vi "Fuzzy_PID.vi"(1 "下限":dbl=330.0 max=349.0 format="%#_13g", 2 "上限":dbl=346.0 min=321.0, 3 "起始值":dbl) -> (0 "调整值":dbl format="%_6g")   [LabVIEW 2016]
uses:
  <vilib>/addons/control/pid/pid.llb/PID (DBL).vi
  <vilib>/addons/Fuzzy Logic/FL Fuzzy Controller (MIMO).vi
  <vilib>/addons/control/pid/NI_PID_pid.lvlib
  <vilib>/addons/Fuzzy Logic/NI_Fuzzy_Logic_API.lvlib
panel:
  out "波形图表":cluster{dbl, "期望值":dbl}(graph)
  out "输入值":dbl
  out "误差变化率":dbl
  out "误差":dbl
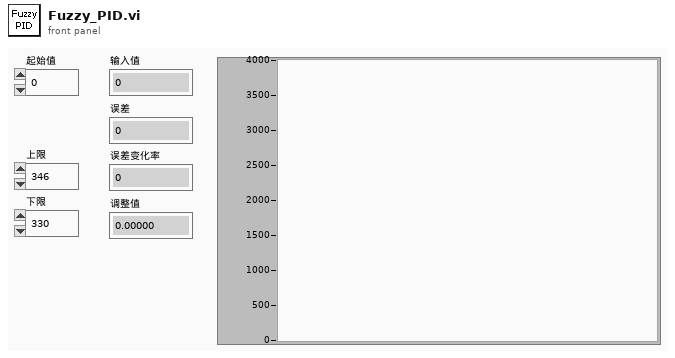
[diagram p1: front panel]
types:
  T1 = typedef "NI_Fuzzy_Logic_API.lvlib/FL System.ctl" = cluster{"input variables":T2[], "output variables":T2[], "rules":T5[], "defuzzification method":T11, "description":string, "user MF interpolating polynomials":T12[]}
  T2 = typedef "NI_Fuzzy_Logic_API.lvlib/FL Variable.ctl" = cluster{"name":string, "range":dbl[], "MFs":T3[]}
  T3 = typedef "NI_Fuzzy_Logic_API.lvlib/FL Membership Function.ctl" = cluster{"name":string, "shape":T4, "points":dbl[], "color":u32, "user-defined shape index":i32}
  T4 = typedef "NI_Fuzzy_Logic_API.lvlib/FL Membership Function Shape.ctl" = u16
  T5 = typedef "NI_Fuzzy_Logic_API.lvlib/FL Rule.ctl" = cluster{"antecedents":T6[], "antecedent connective":T8, "consequents":T9[], "consequent implication":T10, "degree of support":dbl}
  T6 = typedef "NI_Fuzzy_Logic_API.lvlib/FL Antecedent.ctl" = cluster{"Var Index":i32, "MF Index":i32, "Cond":T7}
  T7 = typedef "NI_Fuzzy_Logic_API.lvlib/FL Modifier.ctl" = u16
  T8 = typedef "NI_Fuzzy_Logic_API.lvlib/FL Antecedent Connective.ctl" = u16
  T9 = typedef "NI_Fuzzy_Logic_API.lvlib/FL Consequent.ctl" = cluster{"Var Index":i32, "MF Index":i32, "Cond":T7}
  T10 = typedef "NI_Fuzzy_Logic_API.lvlib/FL Consequent Implication.ctl" = u16
  T11 = typedef "NI_Fuzzy_Logic_API.lvlib/FL Defuzzification.ctl" = u16
  T12 = typedef "NI_Fuzzy_Logic_API.lvlib/FL Interpolating polynomials.ctl" = cluster{"X":dbl[], "Y":dbl[], "Y(x) coeff":dbl[][], "X(y) coeff":dbl[][], "Area(y) coeff":dbl[][], "coa_x(y) coeff":dbl[][]}
  T13 = cluster{"[0]":dbl, "[1]":dbl, "[2]":dbl, "[3]":dbl, "[4]":dbl, "[5]":dbl, "[6]":dbl, "[7]":dbl}
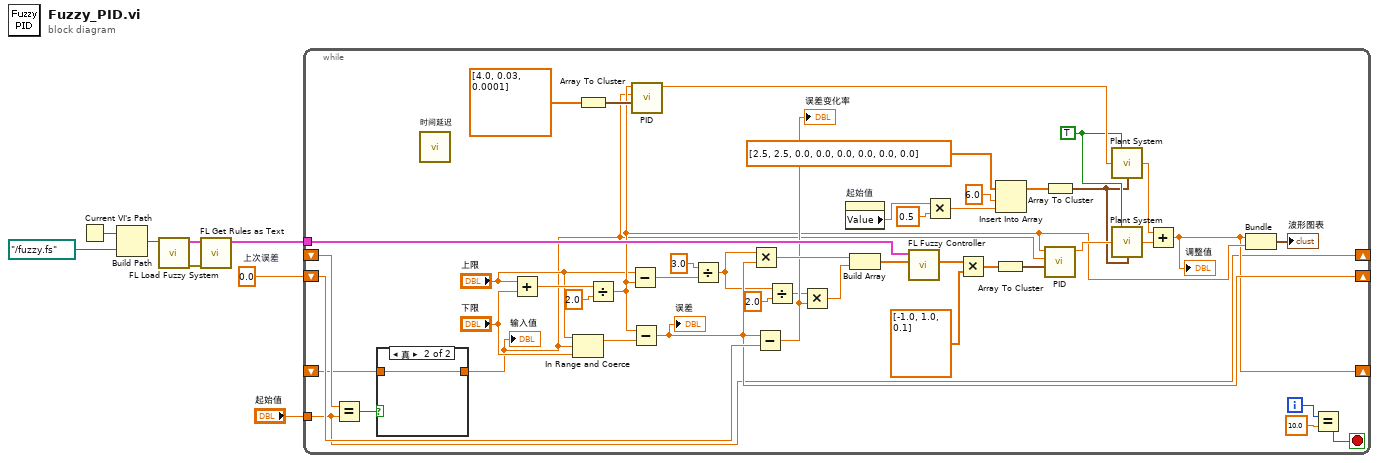
[diagram p0: block diagram]
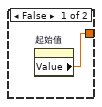
[diagram p2: hidden frame]
diagram:
  w8 = 0.0  # 上次误差
  n1 = Current VI's Path() -> (path=w6:path)
  n2 = Build Path(base path=w6, name or relative path=path "../fuzzy.fs") -> (appended path=w5:path)
  n3 = call <vilib>:"FL Load Fuzzy System.vi"("file path"=w5) -> ("error out"=w3:errorcluster, "fuzzy system out"=w4:T1)  [unwired: 9 in]
  n4 = call <vilib>:"FL Get Rules as Text.vi"("error in (no error)"=w3, "fuzzy system in"=w4) -> ("fuzzy system out"=w2:T1)  [unwired: 7 in, 2 out]
  n5 = while {
    shift-right: [w19] -> _
    shift-left: _ -> [w13]
    shift-right: [w45] -> _
    shift-left: w8 -> [w53]
    tunnel: w2 -> [w47]
    shift-right: [w16] -> _
    shift-left: _ -> [w15]
    tunnel: "起始值" -> [w16]
    i -> [w20]
    stop <- w10 stop-if-true
    w38 = TRUE
    n6 = Equal?(x=w15, y=w16) -> (x = y?=w14:bool)
    n7 = case shown="真" w14 {
      tunnel: w13 -> [_ w56]
      tunnel: [w55 w56] -> w12
      frame False {
        n8 = property on="起始值" class="DigNum (严格)"() -> ("Value"=w55:dbl)  [unwired: 2 in, 2 out]
      }
      frame True {
      }
    }
    "输入值" <- w12
    n9 = call "时间延迟"() -> ()  [unwired: 11 in, 1 out]
    n10 = Add(x="上限", y="下限") -> (x+y=w29:dbl)
    n11 = In Range and Coerce(upper limit="上限", x=w12, lower limit="下限") -> (coerced(x)=w43:dbl)  [unwired: 1 out]
    n12 = Array To Cluster(array=dbl[] [4.0, 0.03, 0.0001]) -> (cluster=w44:cluster{"[0]":dbl, "[1]":dbl, "[2]":dbl})
    n13 = Divide(x=w29, y=2.0) -> (x/y=w25:dbl)
    n14 = Subtract(x="上限", y=w25) -> (x-y=w24:dbl)
    n15 = Subtract(x=w25, y=w43) -> (x-y=w45:dbl)
    "误差" <- w45
    n16 = call-poly <vilib>:"PID.vi"("PID gains"=w44, "process variable"=w12, "setpoint"=w25) -> ("output"=w42:dbl)  [unwired: 7 in, 1 out]
    n17 = Divide(x=3.0, y=w24) -> (x/y=w22:dbl)
    n18 = Multiply(x=w22, y=w45) -> (x*y=w51:dbl)
    n19 = Subtract(x=w45, y=w53) -> (x-y=w46:dbl)
    "误差变化率" <- w46
    n20 = Divide(x=w22, y=2.0) -> (x/y=w26:dbl)
    n21 = Multiply(x=w26, y=w46) -> (x*y=w50:dbl)
    n22 = property on="起始值" class="DigNum (严格)"() -> ("Value"=w11:dbl)  [unwired: 2 in, 2 out]
    n23 = Build Array(w51, w50) -> (w54:dbl[])
    n24 = call-poly <vilib>:"FL Fuzzy Controller.vi"("input values"=w54, "fuzzy system in"=w47) -> ("output values"=w49:dbl[])  [unwired: 5 in, 4 out]
    n25 = Multiply(x=w11, y=0.5 ("initial PV 2")) -> (x*y=w30:dbl)
    n26 = Multiply(x=w49, y=dbl[] [-1.0, 1.0, 0.1]) -> (x*y=w37:dbl[])
    n27 = Array To Cluster(array=w37) -> (cluster=w39:cluster{"[0]":dbl, "[1]":dbl, "[2]":dbl})
    n28 = Insert Into Array(array=dbl[] [2.5, 2.5, 0.0, 0.0, 0.0, 0.0, 0.0, 0.0], index=6.0 ("initial PV 2"), new element=w30) -> (w33:dbl[])
    n29 = Array To Cluster(array=w33) -> (cluster=w32:T13)
    n30 = call-poly <vilib>:"PID.vi"("PID gains"=w39, "process variable"=w12, "setpoint"=w25) -> ("output"=w40:dbl)  [unwired: 7 in, 1 out]
    n31 = call "Plant System.vi"("积分器？"=w38, "设备输入"=w42, "过程参数"=w32) -> ("设备输出"=w35:dbl)  [unwired: 12 in]
    n32 = call "Plant System.vi"("积分器？"=w38, "设备输入"=w40, "过程参数"=w32) -> ("设备输出"=w36:dbl)  [unwired: 12 in]
    n33 = Add(x=w35, y=w36) -> (x+y=w19:dbl)
    "调整值" <- w19
    n34 = Bundle(w19, w25) -> (→"波形图表":cluster{dbl, dbl})  [unwired: 1 in]
    n35 = Equal?(x=w20, y=10.0) -> (x = y?=w10:bool)
  }
